vi "Set_Motors_Brake_All.vi"(8 "error in (no error)":errorcluster) -> (0 "error out":errorcluster)   [LabVIEW 2014]
uses:
  <userlib>/UCSD Robotics Lab/Robotics-Cape/LV/libroboticscape.lvlib
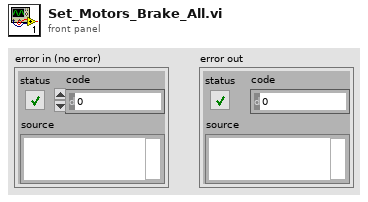
[diagram p1: front panel]
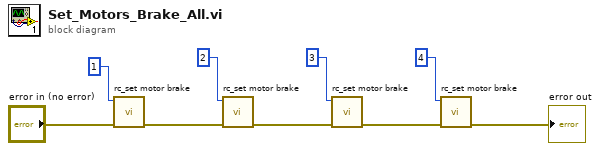
[diagram p0: block diagram]
diagram:
  n1 = call <userlib>:"rc_set motor brake.vi"("error in (no error)"="error in (no error)", "motor"=1) -> ("error out"=w2:errorcluster)  [unwired: 8 in, 1 out]
  n2 = call <userlib>:"rc_set motor brake.vi"("error in (no error)"=w2, "motor"=2) -> ("error out"=w3:errorcluster)  [unwired: 8 in, 1 out]
  n3 = call <userlib>:"rc_set motor brake.vi"("error in (no error)"=w3, "motor"=3) -> ("error out"=w4:errorcluster)  [unwired: 8 in, 1 out]
  n4 = call <userlib>:"rc_set motor brake.vi"("error in (no error)"=w4, "motor"=4) -> ("error out"=→"error out":errorcluster)  [unwired: 8 in, 1 out]
